vi "Item.vi"(8 "error in (no error)":errorcluster, 9 "EventToken":refnum<class "EventToken.lvclass">, 11 "EventBag in":refnum<class "EventBag.lvclass">) -> (0 "error out":errorcluster, 1 "Item found?":bool, 2 "Event":refnum<class "Event.lvclass">, 3 "EventBag out":refnum<class "EventBag.lvclass">)   [LabVIEW 2009, in "EventManagerLibrary.lvlib" / "EventBag.lvclass"]
uses:
  EventBag.lvclass
  EventObject/Event.lvclass
  EventToken/EventToken.lvclass
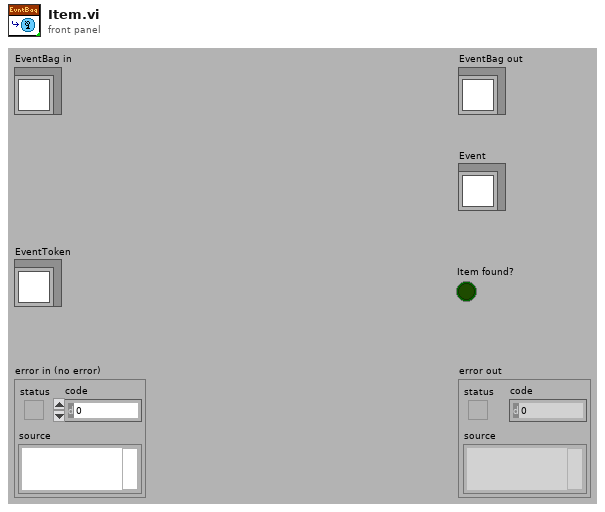
[diagram p1: front panel]
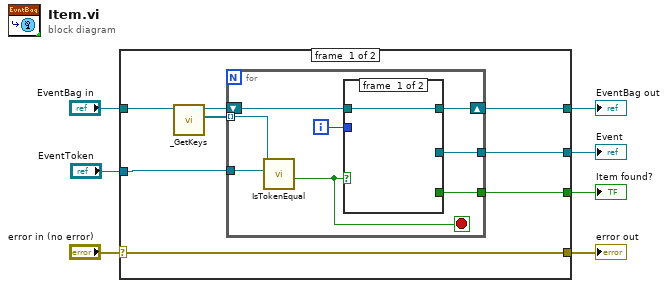
[diagram p0: block diagram]
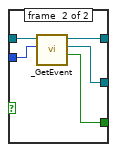
[diagram p2: hidden frame]
diagram:
  n1 = case shown="No Error" "error in (no error)" {
    selector: "error in (no error)" -> [w9 w31]
    tunnel: [w9 w31] -> w6
    tunnel: [w12 w30] -> w4
    tunnel: "EventBag in" -> [w15 w30]
    tunnel: "EventToken" -> [w8 _]
    tunnel: [w11 _] -> w2
    tunnel: [w10 _] -> w1
    frame #0 {
      n2 = call "_GetKeys.vi"("EventBag in"=w15) -> ("Keys"=w14:refnum<class "EventToken.lvclass">[], "EventBag out"=w13:refnum<class "EventBag.lvclass">)  [unwired: 8 in, 1 out]
      n3 = for {
        tunnel: w14 -> [w17] mode=indexing
        shift-right: [w22] -> w12
        shift-left: w13 -> [w23]
        tunnel: [w21] -> w11
        tunnel: [w20] -> w10
        tunnel: w8 -> [w16]
        i -> [w19]
        stop <- w18 stop-if-true
        n4 = call-dynamic "IsTokenEqual.vi"("EventToken"=w16, "EventToken in"=w17) -> ("Is Equal?"=w18:bool)  [unwired: 6 in, 3 out]
        n5 = case shown="True" w18 {
          tunnel: w23 -> [w24 w29]
          tunnel: [w24 w28] -> w22
          tunnel: [_ w27] -> w21
          tunnel: [_ w26] -> w20
          tunnel: w19 -> [_ w25]
          frame #0 {
          }
          frame #1 {
            n6 = call "_GetEvent.vi"("Index"=w25, "EventBag in"=w29) -> ("Item found?"=w26:bool, "Event"=w27:refnum<class "Event.lvclass">, "EventBag out"=w28:refnum<class "EventBag.lvclass">)  [unwired: 6 in, 1 out]
          }
        }
      }
    }
    frame #1 {
    }
  }
  "error out" <- w6
  "EventBag out" <- w4
  "Event" <- w2
  "Item found?" <- w1
